vi "Do.vi"(8 "error in (no error)":errorcluster, 10 "Actor in":refnum<class "Actor.lvclass">, 11 "Publisher Msg":refnum<class "Publisher Msg.lvclass">) -> (0 "error out":errorcluster, 2 "Actor out":refnum<class "Actor.lvclass">)   [LabVIEW 2020, in "Publisher.lvlib" / "Publisher Msg.lvclass"]
doc: "Forward to caller if not Publisher.\nIf Publisher call 'Publisher Do'."
uses:
  Publisher Msg.lvclass
  PPL/HDH.Actor Framework.Core.Actor.lvlibp/1abvi3w/vi.lib/ActorFramework/Actor/Actor.lvclass
  Publisher/Publisher.lvclass
  C:/Current projects/WS/PPL/HDH.Actor Framework.Core.Actor.lvlibp/1abvi3w/vi.lib/ActorFramework/Actor/Actor.lvclass
  Publisher Msg.lvclass/Publisher Msg.ctl
  Read Message Priority.vi
  PPL/HDH.Actor Framework.Core.Actor.lvlibp/1abvi3w/vi.lib/ActorFramework/Actor/Read Caller Enqueuer.vi
  PPL/HDH.Actor Framework.Core.Actor.lvlibp/1abvi3w/vi.lib/ActorFramework/Message Enqueuer/Enqueue.vi
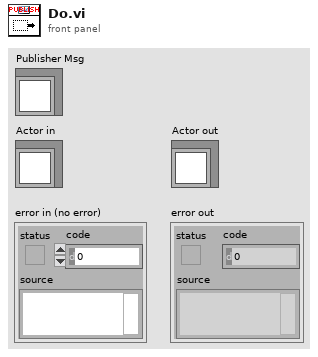
[diagram p1: front panel]
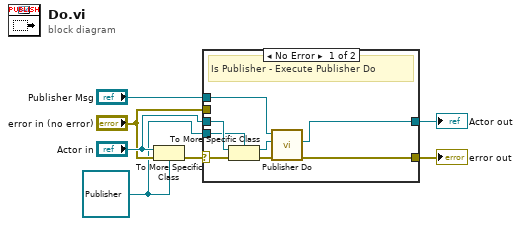
[diagram p0: block diagram]
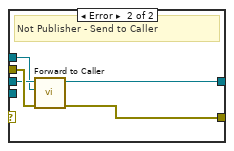
[diagram p2: hidden frame]
diagram:
  w1 = refnum<class "Publisher.lvclass"> refnum ("Actor in")
  n1 = To More Specific Class(target class=w1, reference="Actor in", error in="error in (no error)") -> (error out=w7:errorcluster)  [unwired: 1 out]
  n2 = case shown="No Error" w7 {
    selector: w7 -> [w13 _]
    tunnel: [w10 w17] -> w6
    tunnel: [w8 w18] -> w5
    tunnel: "Actor in" -> [w15 w19]
    tunnel: w1 -> [w14 _]
    tunnel: "error in (no error)" -> [_ w20]
    tunnel: "Publisher Msg" -> [w12 w16]
    frame No Error {
      # "Is Publisher - Execute Publisher Do"
      n3 = To More Specific Class(target class=w14, reference=w15, error in=w13) -> (specific class reference=w9:refnum<class "Publisher.lvclass">, error out=w11:errorcluster)
      n4 = call-dynamic "Publisher Do.vi"("error in (no error)"=w11, "Publisher in"=w9, "Publisher Msg in"=w12) -> ("error out"=w10:errorcluster, "Publisher out"=w8:refnum<class "Publisher.lvclass">)  [unwired: 7 in]
    }
    frame Error {
      # "Not Publisher - Send to Caller"
      n5 = call "Forward to Caller.vi"("error in (no error)"=w20, "Publisher Message"=w16, "Actor in"=w19) -> ("error out"=w17:errorcluster, "Actor out"=w18:refnum<class "Actor.lvclass">)  [unwired: 7 in]
    }
  }
  "error out" <- w6
  "Actor out" <- w5
